vi "Set Report Path.vi"(8 "error in (no error)":errorcluster, 10 "Path":path, 11 "Report Generator In":refnum<class "Report Generator.lvclass">) -> (0 "error out":errorcluster, 3 "Report Generator Out":refnum<class "Report Generator.lvclass">)   [LabVIEW 2020, in "Report Generator.lvclass"]
uses:
  Report Generator.lvclass
  C:/Git/astemes-lunit/source/Application Framework/Process Classes/Process/Process.lvclass
  Report Classes/Plain Text Report/Plain Text Report.lvclass
  C:/Git/astemes-lunit/source/Framework/Report Classes/Test Report/Test Report.lvclass
  Report Classes/Test Report/Test Report.lvclass/Test Report.ctl
  Application Framework/Process Classes/Process/Process.lvclass/Process.ctl
  Report Classes/XML Report/XML Report.lvclass
  <vilib>/Utility/error.llb/Error Cluster From Error Code.vi
  <vilib>/ErrorRing/Error Ring.xnode
  Application Framework/Process Classes/Process/Process.lvclass
  Report Classes/Test Report/Test Report.lvclass
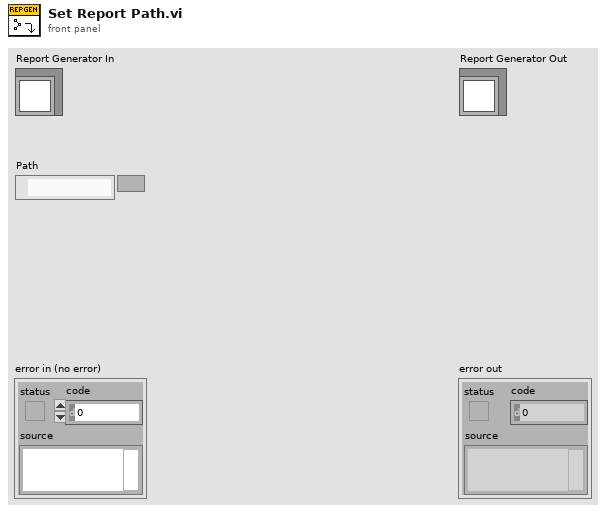
[diagram p1: front panel]
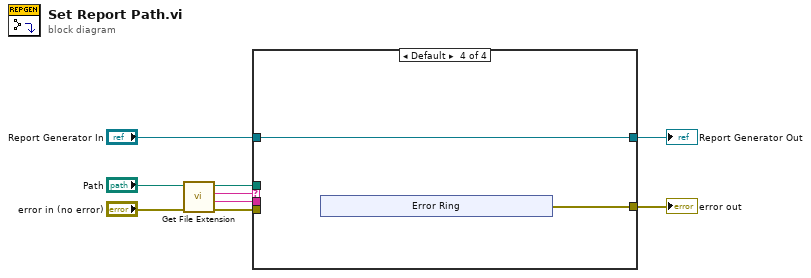
[diagram p0: block diagram]
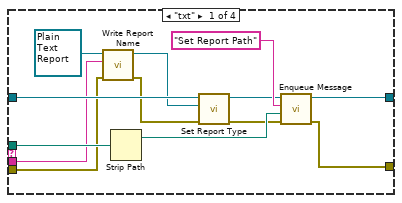
[diagram p2: hidden frame]
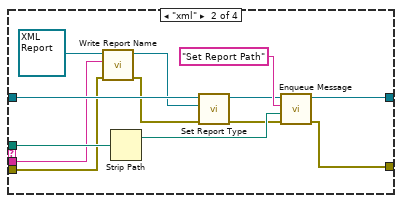
[diagram p3: hidden frame]
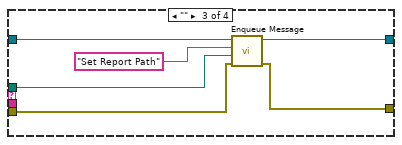
[diagram p4: hidden frame]
diagram:
  n1 = call <vilib>:"Get File Extension.vi"("error in (no error)"="error in (no error)", "file"="Path") -> ("error out"=w2:errorcluster, "filename without extension"=w3:string, "lowercase file extension"=w4:string, "dup file"=w1:path)  [unwired: 5 in, 1 out]
  n2 = case shown="Default" w4 {
    tunnel: [w10 w24 w38 w43] -> w7
    tunnel: "Report Generator In" -> [w17 w31 w40 w42]
    tunnel: w3 -> [w14 w28 _ _]
    tunnel: w2 -> [w13 w27 w37 _]
    tunnel: w1 -> [w21 w34 w36 _]
    tunnel: [w19 w32 w39 w42] -> w8
    frame "txt" {
      n3 = call "Write Report Name.vi"("error in (no error)"=w13, "Report Name"=w14, "Report In"=refnum<class "Plain Text Report.lvclass"> refnum ("Plain Text Report.lvclass")) -> ("error out"=w12:errorcluster, "Report Out"=w15:refnum<class "Plain Text Report.lvclass">)  [unwired: 7 in]
      n4 = Strip Path(path=w21) -> (stripped path=w20:path)  [unwired: 1 out]
      n5 = call "Set Report Type.vi"("error in (no error)"=w12, "Test Report"=w15, "Report Generator In"=w17) -> ("error out"=w11:errorcluster, "Report Generator Out"=w16:refnum<class "Report Generator.lvclass">)  [unwired: 7 in]
      n6 = call "Enqueue Message.vi"("error in (no error)"=w11, "Message Data"=w20, "Message"="Set Report Path", "Process In"=w16) -> ("error out"=w10:errorcluster, "Process Out"=w19:refnum<class "Report Generator.lvclass">)  [unwired: 6 in]
    }
    frame "xml" {
      n7 = call "Write Report Name.vi"("error in (no error)"=w27, "Report Name"=w28, "Report In"=refnum<class "XML Report.lvclass"> refnum ("XML Report.lvclass")) -> ("error out"=w26:errorcluster, "Report Out"=w29:refnum<class "XML Report.lvclass">)  [unwired: 7 in]
      n8 = Strip Path(path=w34) -> (stripped path=w33:path)  [unwired: 1 out]
      n9 = call "Set Report Type.vi"("error in (no error)"=w26, "Test Report"=w29, "Report Generator In"=w31) -> ("error out"=w25:errorcluster, "Report Generator Out"=w30:refnum<class "Report Generator.lvclass">)  [unwired: 7 in]
      n10 = call "Enqueue Message.vi"("error in (no error)"=w25, "Message Data"=w33, "Message"="Set Report Path", "Process In"=w30) -> ("error out"=w24:errorcluster, "Process Out"=w32:refnum<class "Report Generator.lvclass">)  [unwired: 6 in]
    }
    frame "" {
      n11 = call "Enqueue Message.vi"("error in (no error)"=w37, "Message Data"=w36, "Message"="Set Report Path", "Process In"=w40) -> ("error out"=w38:errorcluster, "Process Out"=w39:refnum<class "Report Generator.lvclass">)  [unwired: 6 in]
    }
    frame Default {
      n12 = xnode "Error Ring"() -> ("error out"=w43:errorcluster)
    }
  }
  "error out" <- w7
  "Report Generator Out" <- w8
